vi "FloatToGPS.vi"(1 "数字":dbl) -> (0 "string":string)   [LabVIEW 2018]
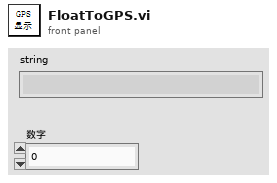
[diagram p1: front panel]
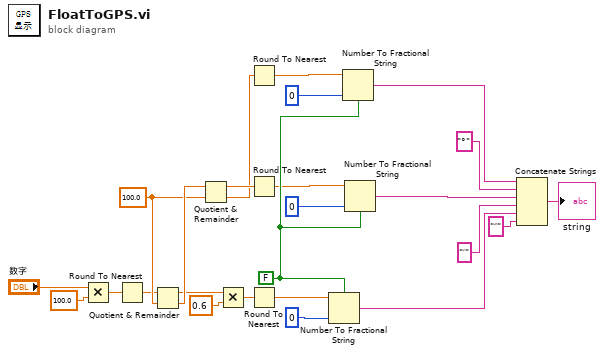
[diagram p0: block diagram]
diagram:
  w20 = FALSE ("使用系统小数点(T)")
  w21 = 100.0 ("y")
  n1 = Multiply(x="数字", y=100.0) -> (x*y=w23:dbl)
  n2 = Round To Nearest(number=w23) -> (nearest integer value=w1:dbl)
  n3 = Quotient & Remainder(x=w1, y=w21) -> (x-y*floor(x/y)=w19:dbl, floor(x/y)=w22:dbl)
  n4 = Quotient & Remainder(x=w22, y=w21) -> (x-y*floor(x/y)=w5:dbl, floor(x/y)=w3:dbl)
  n5 = Multiply(x=w19, y=0.6) -> (x*y=w7:dbl)
  n6 = Round To Nearest(number=w3) -> (nearest integer value=w2:dbl)
  n7 = Round To Nearest(number=w5) -> (nearest integer value=w4:dbl)
  n8 = Round To Nearest(number=w7) -> (nearest integer value=w6:dbl)
  n9 = Number To Fractional String(use system decimal point (T)=w20, number=w6, precision (6)=i16 0 ("精度(6)")) -> (F-format string=w13:string)  [unwired: 1 in]
  n10 = Number To Fractional String(use system decimal point (T)=w20, number=w2, precision (6)=i16 0 ("精度(6)")) -> (F-format string=w17:string)  [unwired: 1 in]
  n11 = Number To Fractional String(use system decimal point (T)=w20, number=w4, precision (6)=i16 0 ("精度(6)")) -> (F-format string=w15:string)  [unwired: 1 in]
  n12 = Concatenate Strings(w17, "°", w15, "′", w13, "″") -> (→"string":string)
